vi "Tri_EmailExpedition.vi"() -> ()   [LabVIEW 2020]
uses:
  Modules/Fonction Standard/Fichier ou dossier/Cluster des Chemins.ctl
panel:
  in  "Article":string="S122.0071 CARINA AVEC FILTRE FERRITE"
  out "Tab_Email_expedition":string[](array[string])
  in  "Tableau Config email":string[][](array[string])
  # "Produit complet ou division"
  # "email fin d'emballage"
  # "present"
  # "email de remplacement si absent"
  # "Email client en copie"
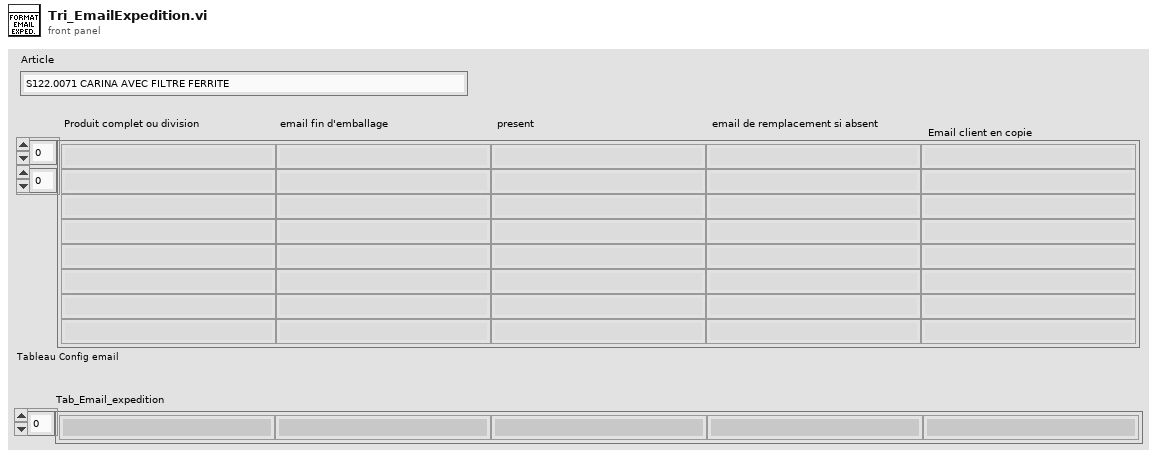
[diagram p1: front panel]
types:
  T1 = typedef "Cluster des Chemins.ctl" = cluster{" Admin-réseau ":path, " XML-Réseau":path, " Résultat tests-Réseau":path, " Archive prôbleme-Réseau":path, " Archive Test  Local":path}
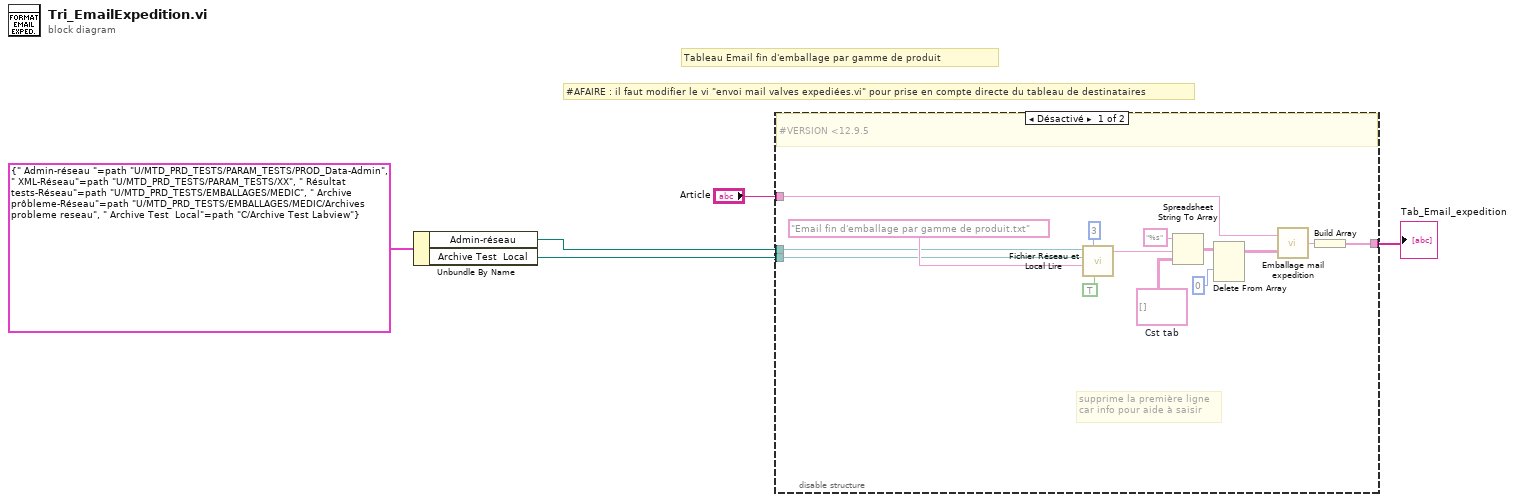
[diagram p0: block diagram]
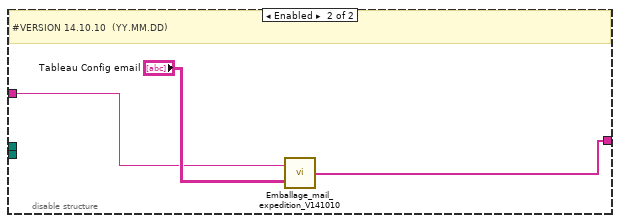
[diagram p2: hidden frame]
diagram:
  # "#AFAIRE : il faut modifier le vi \"envoi mail valves expediées.vi\" pour prise en compte directe du tableau de destinataires"
  # "Tableau Email fin d'emballage par gamme de produit"
  n1 = Unbundle By Name(T1 {" Admin-réseau "=path "U:/MTD_PRD_TESTS/PARAM_TESTS/PROD_Data-Admin", " XML-Réseau"=path "U:/MTD_PRD_TESTS/PARAM_TESTS/XX", " Résultat tests-Réseau"=path "U:/MTD_PRD_TESTS/EMBALLAGES/MEDIC", " Archive prôbleme-Réseau"=path "U:/MTD_PRD_TESTS/EMBALLAGES/MEDIC/Archives probleme reseau", " Archive Test  Local"=path "C:/Archive Test Labview"} ("Chemins-News")) -> ("Admin-réseau"=w4:path, "Archive Test  Local"=w3:path)
  n2 = disable-structure shown="Désactivé" {
    disable-tunnel: w4 -> [w10 _]
    disable-tunnel: w3 -> [w9 _]
    disable-tunnel: [w7 w20] -> w2
    disable-tunnel: "Article" -> [w6 w21]
    frame Disabled {
      w16 = string[][] []  # Cst tab
      # "supprime la première ligne\ncar info pour aide à saisir"
      # "#VERSION <12.9.5"
      n3 = call "Fichier Réseau et Local Lire .vi"("reseau prioritaire ?"=TRUE, "nbr de sous dossier"=3, "Nom fichier"="Email fin d'emballage par gamme de produit.txt", "Dossier Local"=w9, "Fichier ou dossier Reseau"=w10) -> ("Texte"=w12:string)  [unwired: 2 in, 3 out]
      n4 = Spreadsheet String To Array(format string="%s", spreadsheet string=w12, array type (2D Dbl)=w16) -> (array=w14:string[][])  [unwired: 1 in]
      n5 = Delete From Array(array=w14, index (row)=0) -> (array with subset deleted=w11:string[][])  [unwired: 2 in, 1 out]
      n6 = call "Emballage mail expedition.vi"("Tableau mail expedition"=w11, "Article"=w6) -> ("Email expedition"=w8:string)
      n7 = Build Array(w8) -> (w7:string[])
    }
    frame Enabled {
      # "#VERSION 14.10.10  (YY.MM.DD)"
      n8 = call "Emballage_mail_expedition_V141010.vi"("Tableau Config email"="Tableau Config email", "Article"=w21) -> ("Tab_Email_expedition"=w20:string[])
    }
  }
  "Tab_Email_expedition" <- w2
